vi "Raw UTF-16LE String to Raw UTF-8 String.vi"(6 "error in":errorcluster, 9 "Raw UTF-16LE String":T2) -> (1 "Raw UTF-8 String":T1, 4 "error out":errorcluster)   [LabVIEW 2020, in "G-Unicode.lvlib"]
uses:
  G-Unicode.lvlib
  Types/Raw UTF-16LE String.ctl
  Types/Raw UTF-8 String.ctl
  kernel32.dll
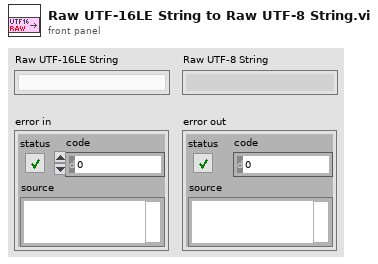
[diagram p1: front panel]
types:
  T1 = typedef "G-Unicode.lvlib/Raw UTF-8 String.ctl" = string
  T2 = typedef "G-Unicode.lvlib/Raw UTF-16LE String.ctl" = string
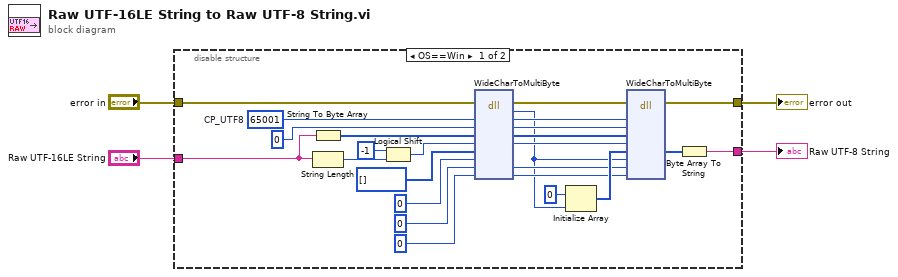
[diagram p0: block diagram]
diagram:
  n1 = disable-structure shown="OS==Win" {
    disable-tunnel: "error in" -> [w26 w31]
    disable-tunnel: "Raw UTF-16LE String" -> [w24 w30]
    disable-tunnel: [w15 w31] -> w2
    disable-tunnel: [w6 w30] -> w1
    frame condition #0 (active) {
      w29 = u32 65001  # CP_UTF8
      n2 = String To Byte Array(string=w24) -> (unsigned byte array=w25:u8[])
      n3 = String Length(string=w24) -> (length=w23:i32)
      n4 = Logical Shift(y=i16 -1, x=w23) -> (x << y=w21:i32)
      n5 = dll-call lib="kernel32.dll" fn="WideCharToMultiByte"(error in=w26, "codePage"=w29, "dwFlags"=u32 0, "lpWideCharStr"=w25, "cchWideChar"=w21, "pMultiByteStr"=u8[] [], "cbMultiByte"=0, "lpDefaultChar"=u8 0, "lpUsedDefaultChar"=0) -> (error out=w16:errorcluster, "return type"=w5:i32, "codePage"=w14:u32, "dwFlags"=w13:u32, "lpWideCharStr"=w12:u8[], "cchWideChar"=w11:i32, "lpDefaultChar"=w9:u8, "lpUsedDefaultChar"=w8:i32)  [unwired: 4 in, 1 out]
      n6 = Initialize Array(u8 0 ("dwFlags"), w5) -> (w10:u8[])
      n7 = dll-call lib="kernel32.dll" fn="WideCharToMultiByte"(error in=w16, "codePage"=w14, "dwFlags"=w13, "lpWideCharStr"=w12, "cchWideChar"=w11, "pMultiByteStr"=w10, "cbMultiByte"=w5, "lpDefaultChar"=w9, "lpUsedDefaultChar"=w8) -> (error out=w15:errorcluster, "pMultiByteStr"=w7:u8[])  [unwired: 9 in, 2 out]
      n8 = Byte Array To String(unsigned byte array=w7) -> (string=w6:string)
    }
    frame condition #1 {
    }
  }
  "error out" <- w2
  "Raw UTF-8 String" <- w1
